vi "Lockin check on.vi"(11 "VISA resource name":refnum<visa-resource-name>="GPIB0::9::INSTR") -> (2 "ready?":bool, 3 "VISA resource name out":refnum<visa-resource-name>)   [LabVIEW 2012, in "SR830.lvlib"]
doc: "Checks to see if the SR830 lock-in amplifier is available or not by requesting its device ID string."
uses:
  SR830.lvlib
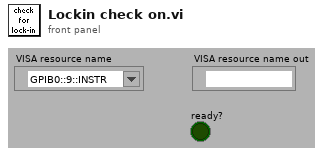
[diagram p1: front panel]
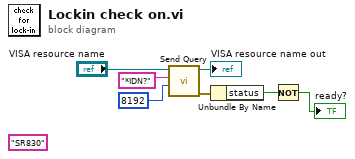
[diagram p0: block diagram]
diagram:
  (unwired) "SR830" ("name (unnamed)")
  n1 = call "Send Query.vi"("Bytes Count"=8192 ("byte count"), "write buffer"="*IDN?" ("data"), "VISA resource name"="VISA resource name") -> ("error out"=w2:errorcluster, "VISA resource name out"=→"VISA resource name out":refnum<visa-resource-name>)  [unwired: 6 in, 1 out]
  n2 = Unbundle By Name(w2) -> ("status"=w7:bool)
  n3 = Not(x=w7) -> (.not. x?=→"ready?":bool)
